vi "Read End-of-File.vi"(5 "Username":string, 6 "Password":string, 7 "Address":string, 8 "Error In":errorcluster) -> (0 "Error Out":errorcluster)   [LabVIEW 2018, in "Tests.lvlib" / "Channel.lvlib"]
uses:
  Channel.lvlib
  src/Toolkit/Channel/Channel.lvclass/Channel.ctl
  src/Toolkit/Session/Session.lvclass/Session.ctl
  src/Toolkit/SSH/SSH.lvclass/SSH.ctl
  src/Toolkit/Session/Utility/Read Shared Library.vi
  src/Toolkit/SSH/Utility/Read Shared Library.vi
  src/Toolkit/Support/Check Status.vi
  <vilib>/addons/_JKI Toolkits/Caraya/classes/Test/Test.lvclass
  <vilib>/addons/_JKI Toolkits/Caraya/classes/Assert/Assert.lvclass
  src/Toolkit/Channel/Channel.lvclass
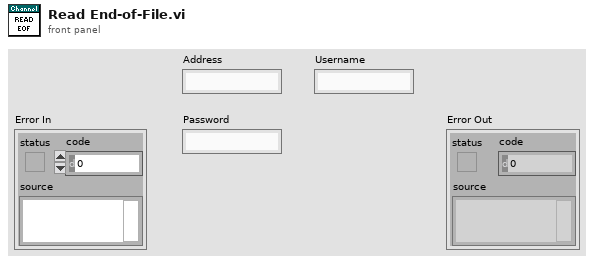
[diagram p1: front panel]
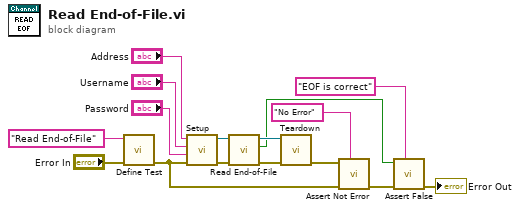
[diagram p0: block diagram]
diagram:
  n1 = call <vilib>:"Define Test.vi"("error in (no error)"="Error In", "Label (VI Title)"="Read End-of-File") -> ("error out"=w13:errorcluster)  [unwired: 9 in]
  n2 = call "Setup.vi"("Error In"=w13, "Password"="Password", "Username"="Username", "Address"="Address") -> ("Error Out"=w5:errorcluster, "Channel"=w8:refnum<class "Channel.lvclass">)  [unwired: 6 in]
  n3 = call "Read End-of-File.vi"("Error In"=w5, "Channel In"=w8) -> ("Error Out"=w6:errorcluster, "End-of-File?"=w2:bool, "Channel Out"=w7:refnum<class "Channel.lvclass">)  [unwired: 7 in]
  n4 = call "Teardown.vi"("Error In"=w6, "Channel"=w7) -> ("Error Out"=w9:errorcluster)  [unwired: 9 in]
  n5 = call <vilib>:"Assert Not Error.vi"("Label"="No Error", "error in (no error)"=w13, "Not Error?"=w9) -> ("error out"=w4:errorcluster)  [unwired: 8 in]
  n6 = call <vilib>:"Assert False.vi"("Label"="EOF is correct", "error in (no error)"=w4, "False?"=w2) -> ("error out"=→"Error Out":errorcluster)  [unwired: 8 in]
